vi "Write Context.vi"(8 "error in (no error)":errorcluster, 10 "Debug Process.lvclass":refnum<class "Debug Process.lvclass">, 11 "Debug View In":refnum<class "Debug View.lvclass">) -> (0 "error out":errorcluster, 3 "Debug View Out":refnum<class "Debug View.lvclass">)   [LabVIEW 2020, in "Debug View.lvclass"]
uses:
  Debug View.lvclass
  Process/Debug Process.lvclass
  Debug View.lvclass/Debug View.ctl
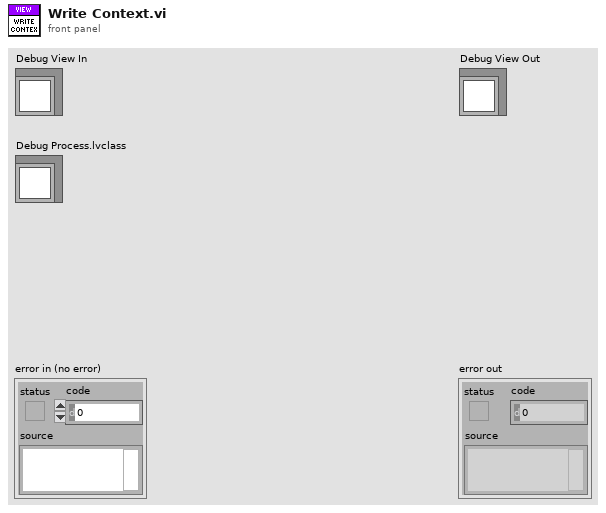
[diagram p1: front panel]
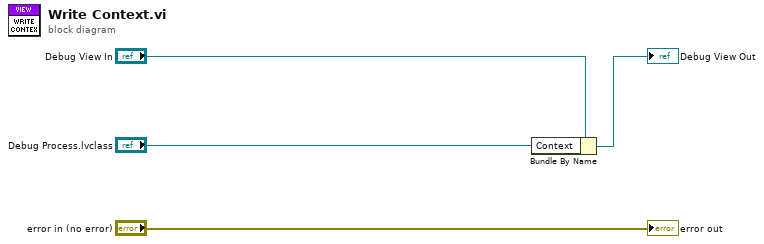
[diagram p0: block diagram]
diagram:
  n1 = Bundle By Name(cluster="Debug View In", "Context"="Debug Process.lvclass") -> (→"Debug View Out":refnum<class "Debug View.lvclass">)
  "error out" <- "error in (no error)"
